vi "Stop.vi"(8 "error in (no error)":errorcluster, 10 "Message in":refnum<class "StopMessage.lvclass">, 11 "RSA in":refnum<class "RSA.lvclass">) -> (0 "error out":errorcluster, 3 "RSA out":refnum<class "RSA.lvclass">)   [LabVIEW 2012, in "RSA.lvclass"]
doc: "This member function is called when the statemachine in the run.vi receives an 'stop' command. It relays the message to all observers of the component.\n\nOverride this member function in your derived class if you need additional stop functionality (but don't forget to call the parent method)."
uses:
  RSA.lvclass
  <vilib>/Distrio/Murmex/StopMessage/StopMessage.lvclass
  <vilib>/Distrio/Murmex/Murmex/Murmex.lvclass
  RSA.lvclass/RSA.ctl
  <vilib>/Utility/file.llb/Write To Spreadsheet File (DBL).vi
panel:
  # "This method is called when the STOP\ntrigger is sent. \n\nOverride this method when your component needs to\nrespond to this trigger. \n\nCall parent for proper implementation"
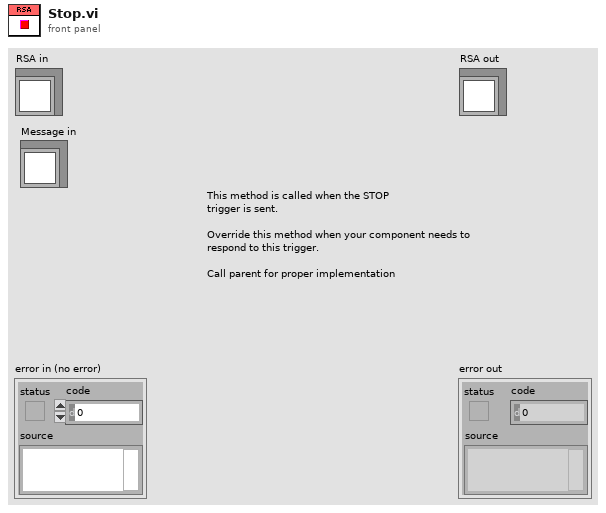
[diagram p1: front panel]
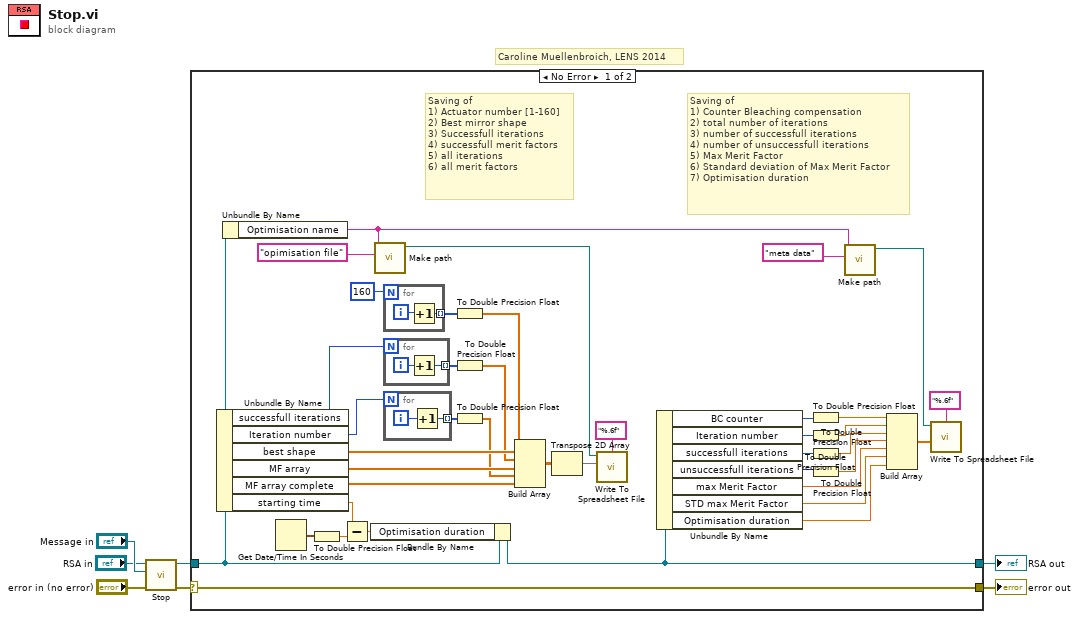
[diagram p0: block diagram]
diagram:
  # "Caroline Muellenbroich, LENS 2014"
  n1 = call-parent "Stop.vi"("error in (no error)"="error in (no error)", "Message in"="Message in", "Murmex in"="RSA in") -> ("error out"=w4:errorcluster, "Murmex out"=w2:refnum<class "RSA.lvclass">)  [unwired: 7 in]
  n2 = case shown="No Error" w4 {
    selector: w4 -> [w47 w54]
    tunnel: [w47 w54] -> w3
    tunnel: w2 -> [w28 w55]
    tunnel: [w25 w55] -> w1
    frame No Error {
      # "Saving of\n1) Counter Bleaching compensation\n2) total number of iterations\n3) number of successfull iterations\n4) number of unsuccessfull iterations\n5) Max Merit Factor\n6) Standard deviation of Max Merit Factor\n7) Optimisation duration"
      # "Saving of\n1) Actuator number [1-160]\n2) Best mirror shape\n3) Successfull iterations\n4) successfull merit factors\n5) all iterations\n6) all merit factors"
      n3 = Unbundle By Name(w28) -> ("successfull iterations"=w38:i32, "Iteration number"=w35:i32, "best shape"=w34:dbl[], "MF array"=w32:dbl[], "MF array complete"=w30:dbl[], "starting time"=w45:dbl)
      n4 = Unbundle By Name(w28) -> ("Optimisation name"=w10:string)
      n5 = Get Date/Time In Seconds() -> (seconds since 1Jan1904=w46:timestamp)
      n6 = To Double Precision Float(number=w46) -> (double precision float=w44:dbl)
      n7 = Subtract(x=w45, y=w44) -> (x-y=w43:dbl)
      n8 = Bundle By Name(cluster=w28, "Optimisation duration"=w43) -> (w25:refnum<class "RSA.lvclass">)
      n9 = call "Make path.vi"("what?"="opimisation file" ("string"), "name"=w10) -> ("path"=w26:path)  [unwired: 9 in]
      n10 = for {
        N: 160 -> [_]
        tunnel: [w52] -> w41 mode=indexing
        i -> [w53]
        n11 = Increment(x=w53) -> (x+1=w52:i32)
      }
      n12 = for {
        N: w38 -> [_]
        tunnel: [w48] -> w37 mode=indexing
        i -> [w49]
        n13 = Increment(x=w49) -> (x+1=w48:i32)
      }
      n14 = for {
        N: w35 -> [_]
        tunnel: [w50] -> w39 mode=indexing
        i -> [w51]
        n15 = Increment(x=w51) -> (x+1=w50:i32)
      }
      n16 = To Double Precision Float(number=w41) -> (double precision float=w40:dbl[])
      n17 = To Double Precision Float(number=w37) -> (double precision float=w33:dbl[])
      n18 = To Double Precision Float(number=w39) -> (double precision float=w31:dbl[])
      n19 = Build Array(w40, w34, w33, w32, w31, w30) -> (w36:dbl[][])
      n20 = Transpose 2D Array(2D array=w36) -> (transposed array=w24:dbl[][])
      n21 = call-poly <vilib>:"Write To Spreadsheet File.vi"("format (%.3f)"="%.6f", "2D data"=w24, "file path (dialog if empty)"=w26) -> ()  [unwired: 3 in, 3 out]
      n22 = Unbundle By Name(w25) -> ("BC counter"=w23:i32, "Iteration number"=w22:i32, "successfull iterations"=w21:i32, "unsuccessfull iterations"=w20:i32, "max Merit Factor"=w15:dbl, "STD max Merit Factor"=w14:dbl, "Optimisation duration"=w13:dbl)
      n23 = To Double Precision Float(number=w23) -> (double precision float=w19:dbl)
      n24 = To Double Precision Float(number=w22) -> (double precision float=w18:dbl)
      n25 = To Double Precision Float(number=w21) -> (double precision float=w17:dbl)
      n26 = To Double Precision Float(number=w20) -> (double precision float=w16:dbl)
      n27 = call "Make path.vi"("what?"="meta data" ("string"), "name"=w10) -> ("path"=w8:path)  [unwired: 9 in]
      n28 = Build Array(w19, w18, w17, w16, w15, w14, w13) -> (w11:dbl[])
      n29 = call-poly <vilib>:"Write To Spreadsheet File.vi"("format (%.3f)"="%.6f", "1D data"=w11, "file path (dialog if empty)"=w8) -> ()  [unwired: 3 in, 3 out]
    }
    frame Error {
    }
  }
  "error out" <- w3
  "RSA out" <- w1
